vi "Read Manufacturer Name.vi"() -> ()   [LabVIEW 2016]
uses:
  <vilib>/CANopenLib/CANOPEN.llb/CANopen BaudRate.ctl
  <vilib>/userdefined/High Color/nirio_resource_hc.ctl
  <vilib>/FPGAPlugInAG/cRIO-9033/niLvFpga_Open_cRIO-9033.vi
  <vilib>/rvi/interface/common/dynamic/niFpgaDynamicAddResources.vi
  <vilib>/CANopenLib/CANOPEN.llb/CANopen Interface Create.vi
  <vilib>/CANopenLib/CANOPEN.llb/CANopen SDO Create.vi
  <vilib>/CANopenLib/CANOPEN.llb/CANopen SDO Read [STR].vi
  <vilib>/CANopenLib/CANOPEN.llb/CANopen SDO Close.vi
  <vilib>/CANopenLib/CANOPEN.llb/CANopen Interface Close.vi
  <vilib>/rvi/interface/nirviOpenFPGA/nirviOpenFPGA.xnode
  FPGA Bitfiles/project_FPGATarget_FPGAMain_kDJZXzfRsH0.lvbitx
  Program Files (x86)/National Instruments/LabVIEW 2016/examples/robotics/EPOS2 CANOpen Driver/FPGA/FPGA Main.vi
panel:
  out "description":string
  out "Manufacturer Name":string
  in  "interface name":u32(ring) items=["CANopen01", "CANopen02", "CANopen03", "CANopen04", "CANopen05", "CANopen06", "CANopen07", "CANopen08", "CANopen09", "CANopen10", "CANopen11", "CANopen12", "CANopen13", "CANopen14", "CANopen15", "CANopen16", "CANopen17", "CANopen18", "CANopen19", "CANopen20", "CANopen21", "CANopen22", "CANopen23", "CANopen24", "CANopen25", "CANopen26", "CANopen27", "CANopen28", "CANopen29", "CANopen30", "CANopen31", "CANopen32"]
  in  "node-ID (0)":u8=1
  in  "baud rate":T1 items=["1 Mbit/s"=0, "800 kbit/s"=1, "500 kbit/s"=2, "250 kbit/s"=3, "125 kbit/s"=4, "50 kbit/s"=6, "20 kbit/s"=7, "10 kbit/s"=8]
  in  "termination? (F)":bool=TRUE
  out "error out":errorcluster
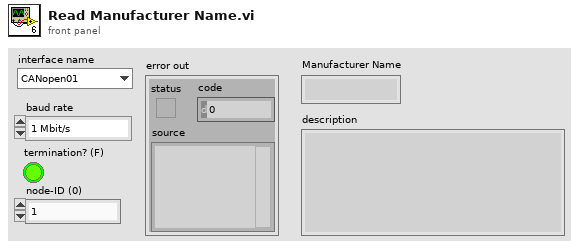
[diagram p1: front panel]
types:
  T1 = typedef "CANopen BaudRate.ctl" = u32
  T2 = typedef "nirio_resource_hc.ctl" = tag
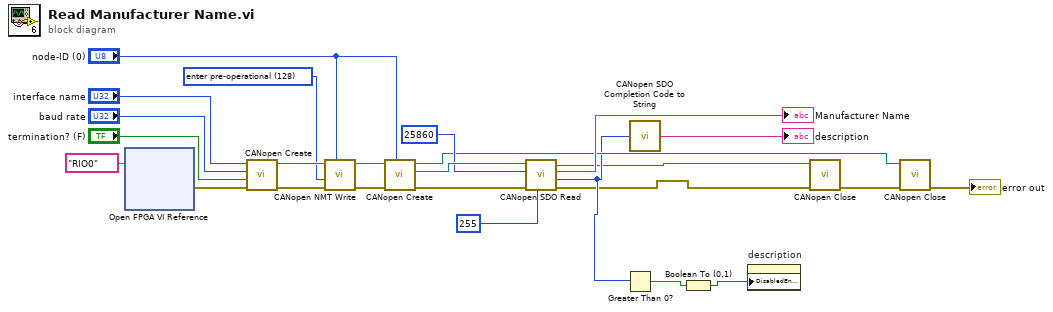
[diagram p0: block diagram]
diagram:
  w21 = u16 128 items=["start remote node"=1, "stop remote node"=2, "enter pre-operational"=128, "reset node"=129, "reset communication"=130] ("command")
  n1 = xnode ("Open FPGA VI Reference")("resource name"=T2 "RIO0") -> ("error out"=w24:errorcluster)  [unwired: 1 in, 1 out]
  n2 = call-poly <vilib>:"CANopen Create.vi"("error in (no error)"=w24, "termination? (F)"="termination? (F)", "baud rate"="baud rate", "interface name"="interface name") -> ("error out"=w23:errorcluster, "interface object out"=w22:refnum<k20>)  [unwired: 6 in]
  n3 = call <vilib>:"CANopen NMT Write.vi"("node-ID (0)"="node-ID (0)", "error in (no error)"=w23, "command"=w21, "interface object in"=w22) -> ("error out"=w9:errorcluster, "interface object out"=w10:refnum<k20>)  [unwired: 6 in]
  n4 = call-poly <vilib>:"CANopen Create.vi"("node-ID"="node-ID (0)", "error in (no error)"=w9, "interface object in"=w10) -> ("error out"=w15:errorcluster, "SDO object out"=w16:refnum<k20>, "interface object out"=w7:refnum<k20>)  [unwired: 6 in]
  n5 = call-poly <vilib>:"CANopen SDO Read.vi"("data size"=u32 255, "error in (no error)"=w15, "object index"=u16 25860, "SDO object in"=w16) -> ("error out"=w1:errorcluster, "completion code"=w6:u32, "string data"=→"Manufacturer Name":string, "SDO object out"=w2:refnum<k20>)  [unwired: 4 in]
  n6 = Greater Than 0?(x=w6) -> (x > 0?=w5:bool)
  n7 = call <vilib>:"CANopen SDO Completion Code to String.vi"("SDO completion code"=w6) -> ("description"=→"description":string)
  n8 = Boolean To (0,1)(Boolean=w5) -> (0, 1=w4:i16)
  n9 = property on="description" class="Str"("DisabledEnum"=w4) -> ()  [unwired: 2 in, 2 out]
  n10 = call-poly <vilib>:"CANopen Close.vi"("error in (no error)"=w1, "SDO object in"=w2) -> ("error out"=w8:errorcluster)  [unwired: 9 in]
  n11 = call-poly <vilib>:"CANopen Close.vi"("error in (no error)"=w8, "interface object in"=w7) -> ("error out"=→"error out":errorcluster)  [unwired: 9 in]
